vi "Reverse Direction.vi"(11 "Direction":i32) -> (3 "Numeric":i32)   [LabVIEW 2014, in "Formics.lvclass"]
uses:
  Formics.lvclass
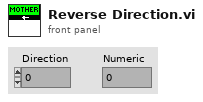
[diagram p1: front panel]
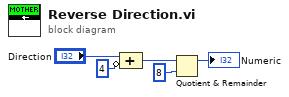
[diagram p0: block diagram]
diagram:
  n1 = Compound Arithmetic op=ADD("Direction", invert 4 ("value")) -> (w3:i32)
  n2 = Quotient & Remainder(x=w3, y=8) -> (x-y*floor(x/y)=→"Numeric":i32)  [unwired: 1 out]
